vi "camera_number.vi"() -> ()   [LabVIEW 2022 SP3]
panel:
  in  "Refresh Button":bool
  in  "4 2":string
  in  "3 2":string caption="3"
  in  "2 2":string
  in  "1 2":string
  out "error out 8":errorcluster
  out "error out 7":errorcluster
  out "error out 6":errorcluster
  out "error out 5":errorcluster
  out "error out":errorcluster
  in  "OK Button 2":bool
  out "error out 2":errorcluster
  out "error out 3":errorcluster
  out "error out 4":errorcluster
  in  "4":string
  in  "3":string
  in  "2":string
  in  "1":string
  # "REFERENCE CHECK"
  # "CAM A"
  # "CAM B"
  # "CAM C"
  # "CAM D"
  # "Refresh"
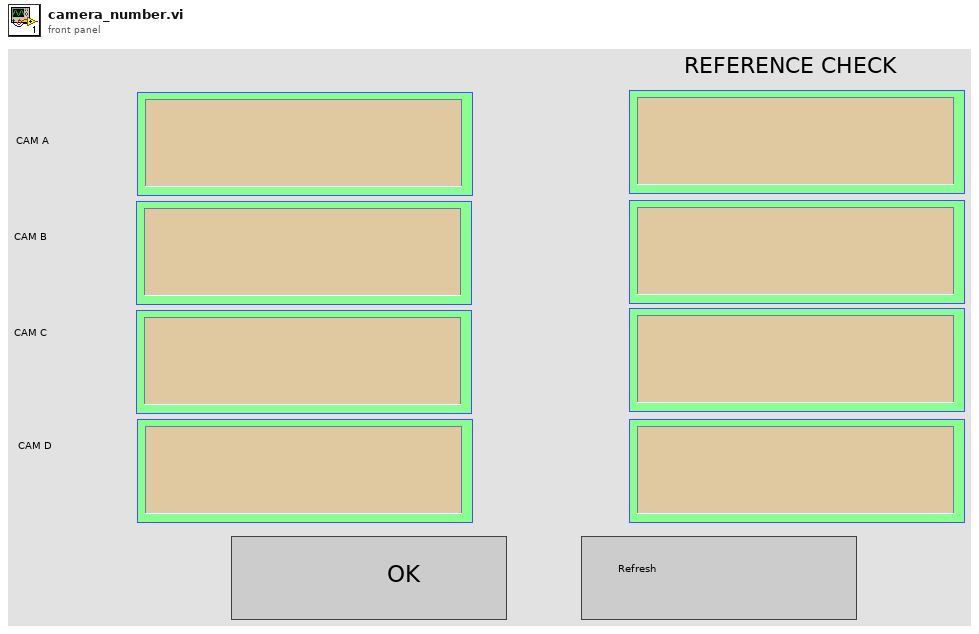
[diagram p1: front panel]
types:
  T1 = enum16{"open", "replace", "create", "open or create", "replace or create", "replace or create with confirmation"}
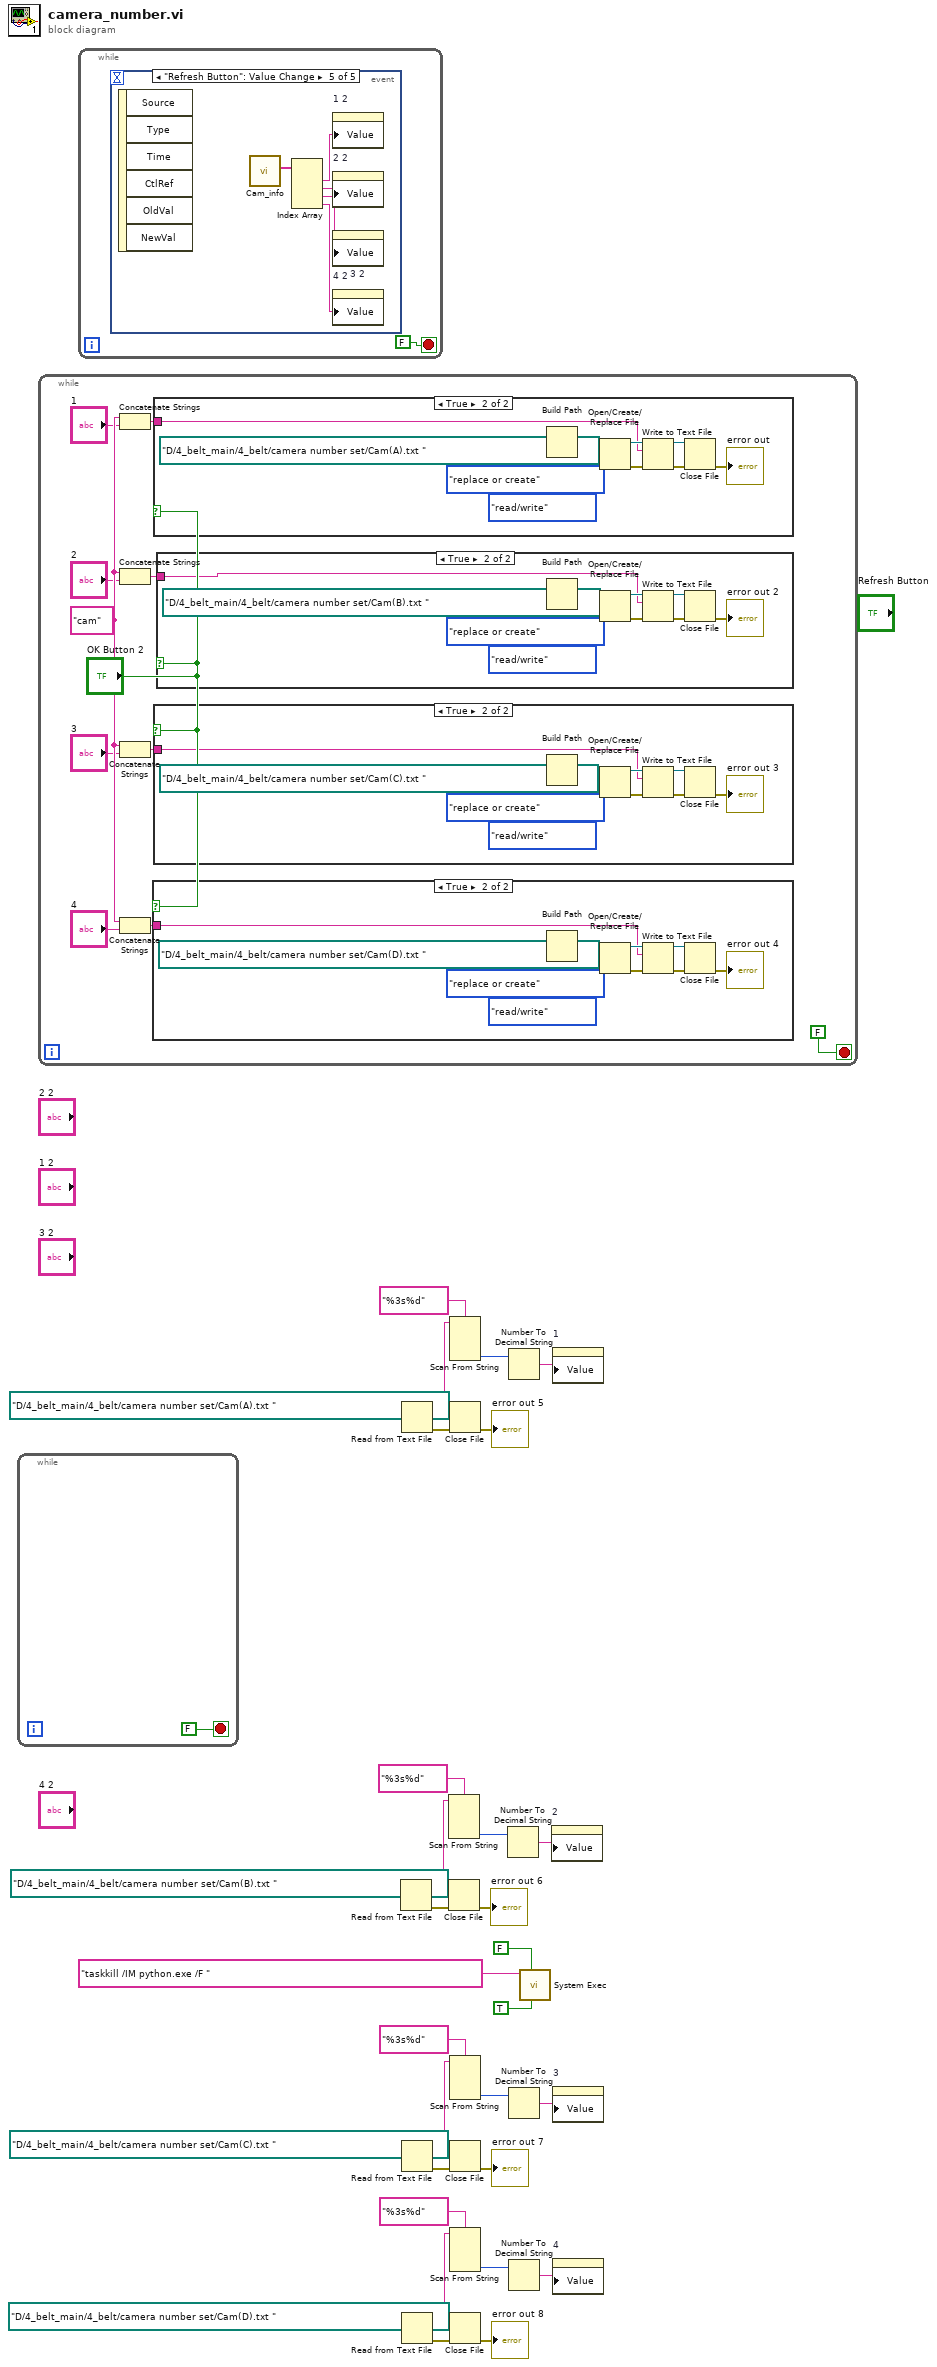
[diagram p0: block diagram]
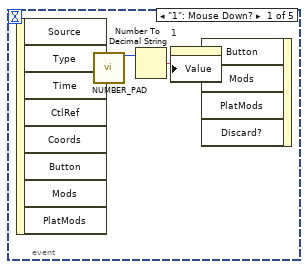
[diagram p2: hidden frame]
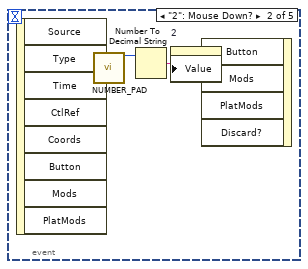
[diagram p3: hidden frame]
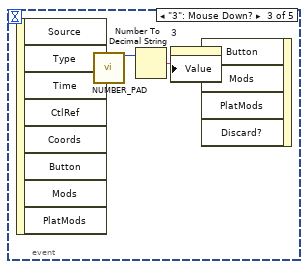
[diagram p4: hidden frame]
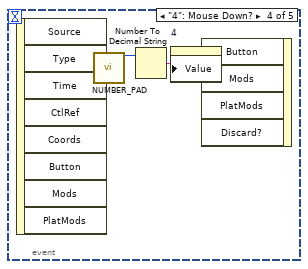
[diagram p5: hidden frame]
diagram:
  n1 = while {
    stop <- FALSE stop-if-true
  }
  n2 = while {
    stop <- FALSE stop-if-true
    w47 = "cam"
    n3 = Concatenate Strings(w47, "1") -> (w46:string)
    n4 = Concatenate Strings(w47, "2") -> (w45:string)
    n5 = Concatenate Strings(w47, "3") -> (w44:string)
    n6 = Concatenate Strings(w47, "4") -> (w43:string)
    n7 = case shown="True" "OK Button 2" {
      tunnel: w43 -> [_ w49]
      frame False {
      }
      frame True {
        n8 = Build Path(name or relative path=path "D:/4_belt_main/4_belt/camera number set/Cam(D).txt " ("base path")) -> (appended path=w57:path)  [unwired: 1 in]
        n9 = Open/Create/Replace File(file path (use dialog)=w57, operation (0:open)=T1."replace or create", access (0:read/write)=enum16{"read/write", "read-only", "write-only"}."read/write") -> (refnum out=w54:refnum<file>, error out=w53:errorcluster)  [unwired: 3 in, 1 out]
        n10 = Write to Text File(file (use dialog)=w54, text=w49, error in=w53) -> (refnum out=w51:refnum<file>, error out=w52:errorcluster)  [unwired: 1 in, 1 out]
        n11 = Close File(refnum=w51, error in=w52) -> (error out=→"error out 4":errorcluster)  [unwired: 1 out]
      }
    }
    n12 = case shown="True" "OK Button 2" {
      tunnel: w46 -> [_ w79]
      frame False {
      }
      frame True {
        n13 = Build Path(name or relative path=path "D:/4_belt_main/4_belt/camera number set/Cam(A).txt " ("base path")) -> (appended path=w87:path)  [unwired: 1 in]
        n14 = Open/Create/Replace File(file path (use dialog)=w87, operation (0:open)=T1."replace or create", access (0:read/write)=enum16{"read/write", "read-only", "write-only"}."read/write") -> (refnum out=w84:refnum<file>, error out=w83:errorcluster)  [unwired: 3 in, 1 out]
        n15 = Write to Text File(file (use dialog)=w84, text=w79, error in=w83) -> (refnum out=w81:refnum<file>, error out=w82:errorcluster)  [unwired: 1 in, 1 out]
        n16 = Close File(refnum=w81, error in=w82) -> (error out=→"error out":errorcluster)  [unwired: 1 out]
      }
    }
    n17 = case shown="True" "OK Button 2" {
      tunnel: w44 -> [_ w59]
      frame False {
      }
      frame True {
        n18 = Build Path(name or relative path=path "D:/4_belt_main/4_belt/camera number set/Cam(C).txt " ("base path")) -> (appended path=w67:path)  [unwired: 1 in]
        n19 = Open/Create/Replace File(file path (use dialog)=w67, operation (0:open)=T1."replace or create", access (0:read/write)=enum16{"read/write", "read-only", "write-only"}."read/write") -> (refnum out=w64:refnum<file>, error out=w63:errorcluster)  [unwired: 3 in, 1 out]
        n20 = Write to Text File(file (use dialog)=w64, text=w59, error in=w63) -> (refnum out=w61:refnum<file>, error out=w62:errorcluster)  [unwired: 1 in, 1 out]
        n21 = Close File(refnum=w61, error in=w62) -> (error out=→"error out 3":errorcluster)  [unwired: 1 out]
      }
    }
    n22 = case shown="True" "OK Button 2" {
      tunnel: w45 -> [_ w69]
      frame False {
      }
      frame True {
        n23 = Build Path(name or relative path=path "D:/4_belt_main/4_belt/camera number set/Cam(B).txt " ("base path")) -> (appended path=w77:path)  [unwired: 1 in]
        n24 = Open/Create/Replace File(file path (use dialog)=w77, operation (0:open)=T1."replace or create", access (0:read/write)=enum16{"read/write", "read-only", "write-only"}."read/write") -> (refnum out=w74:refnum<file>, error out=w73:errorcluster)  [unwired: 3 in, 1 out]
        n25 = Write to Text File(file (use dialog)=w74, text=w69, error in=w73) -> (refnum out=w71:refnum<file>, error out=w72:errorcluster)  [unwired: 1 in, 1 out]
        n26 = Close File(refnum=w71, error in=w72) -> (error out=→"error out 2":errorcluster)  [unwired: 1 out]
      }
    }
  }
  n27 = while {
    stop <- FALSE stop-if-true
    n28 = event shown="[4] \"Refresh Button\": Value Change" {
      selector: _ -> [_ _ _ _ _]
      dyn-events: _ -> [_ _ _ _ _]
      timeout: _ -> [_ _ _ _ _]
      event "1": Mouse Down? {
        n29 = event-data() -> ()  [unwired: 1 in, 8 out]
        n30 = call "NUMBER_PAD.vi"() -> ("number (out)"=w90:i32)  [unwired: 15 in]
        n31 = Number To Decimal String(number=w90) -> (decimal integer string=w89:string)  [unwired: 1 in]
        n32 = property on="1" class="Str"("Value"=w89) -> ()  [unwired: 2 in, 2 out]
        n33 = event-data() -> ()  [unwired: 5 in, 1 out]
      }
      event "2": Mouse Down? {
        n34 = event-data() -> ()  [unwired: 1 in, 8 out]
        n35 = call "NUMBER_PAD.vi"() -> ("number (out)"=w92:i32)  [unwired: 15 in]
        n36 = Number To Decimal String(number=w92) -> (decimal integer string=w91:string)  [unwired: 1 in]
        n37 = property on="2" class="Str"("Value"=w91) -> ()  [unwired: 2 in, 2 out]
        n38 = event-data() -> ()  [unwired: 5 in, 1 out]
      }
      event "3": Mouse Down? {
        n39 = event-data() -> ()  [unwired: 1 in, 8 out]
        n40 = call "NUMBER_PAD.vi"() -> ("number (out)"=w94:i32)  [unwired: 15 in]
        n41 = Number To Decimal String(number=w94) -> (decimal integer string=w93:string)  [unwired: 1 in]
        n42 = property on="3" class="Str"("Value"=w93) -> ()  [unwired: 2 in, 2 out]
        n43 = event-data() -> ()  [unwired: 5 in, 1 out]
      }
      event "4": Mouse Down? {
        n44 = event-data() -> ()  [unwired: 1 in, 8 out]
        n45 = call "NUMBER_PAD.vi"() -> ("number (out)"=w96:i32)  [unwired: 15 in]
        n46 = Number To Decimal String(number=w96) -> (decimal integer string=w95:string)  [unwired: 1 in]
        n47 = property on="4" class="Str"("Value"=w95) -> ()  [unwired: 2 in, 2 out]
        n48 = event-data() -> ()  [unwired: 5 in, 1 out]
      }
      event "Refresh Button": Value Change {
        n49 = event-data() -> ()  [unwired: 1 in, 6 out]
        n50 = call "Cam_info.vi"() -> ("All Cameras"=w101:string[])  [unwired: 10 in, 1 out]
        n51 = Index Array(array=w101) -> (element #1=w100:string, element #2=w99:string, element #3=w98:string, element #4=w97:string)  [unwired: 4 in]
        n52 = property on="1 2" class="Str"("Value"=w100) -> ()  [unwired: 2 in, 2 out]
        n53 = property on="2 2" class="Str"("Value"=w99) -> ()  [unwired: 2 in, 2 out]
        n54 = property on="3 2" class="Str"("Value"=w98) -> ()  [unwired: 2 in, 2 out]
        n55 = property on="4 2" class="Str"("Value"=w97) -> ()  [unwired: 2 in, 2 out]
      }
    }
  }
  n56 = Read from Text File(file (use dialog)=path "D:/4_belt_main/4_belt/camera number set/Cam(B).txt " ("base path")) -> (refnum out=w22:refnum<file>, text=w26:string, error out=w23:errorcluster)  [unwired: 3 in, 1 out]
  n57 = Read from Text File(file (use dialog)=path "D:/4_belt_main/4_belt/camera number set/Cam(A).txt " ("base path")) -> (refnum out=w35:refnum<file>, text=w31:string, error out=w34:errorcluster)  [unwired: 3 in, 1 out]
  n58 = Read from Text File(file (use dialog)=path "D:/4_belt_main/4_belt/camera number set/Cam(C).txt " ("base path")) -> (refnum out=w21:refnum<file>, text=w17:string, error out=w20:errorcluster)  [unwired: 3 in, 1 out]
  n59 = Read from Text File(file (use dialog)=path "D:/4_belt_main/4_belt/camera number set/Cam(D).txt " ("base path")) -> (refnum out=w8:refnum<file>, text=w12:string, error out=w9:errorcluster)  [unwired: 3 in, 1 out]
  n60 = Scan From String(format string="%3s%d", input string=w26) -> (output 2=w28:i32)  [unwired: 5 in, 3 out]
  n61 = Close File(refnum=w22, error in=w23) -> (error out=→"error out 6":errorcluster)  [unwired: 1 out]
  n62 = Scan From String(format string="%3s%d", input string=w31) -> (output 2=w29:i32)  [unwired: 5 in, 3 out]
  n63 = Close File(refnum=w35, error in=w34) -> (error out=→"error out 5":errorcluster)  [unwired: 1 out]
  n64 = Scan From String(format string="%3s%d", input string=w17) -> (output 2=w15:i32)  [unwired: 5 in, 3 out]
  n65 = Close File(refnum=w21, error in=w20) -> (error out=→"error out 7":errorcluster)  [unwired: 1 out]
  n66 = Scan From String(format string="%3s%d", input string=w12) -> (output 2=w14:i32)  [unwired: 5 in, 3 out]
  n67 = Close File(refnum=w8, error in=w9) -> (error out=→"error out 8":errorcluster)  [unwired: 1 out]
  n68 = Number To Decimal String(number=w28) -> (decimal integer string=w2:string)  [unwired: 1 in]
  n69 = Number To Decimal String(number=w29) -> (decimal integer string=w1:string)  [unwired: 1 in]
  n70 = Number To Decimal String(number=w15) -> (decimal integer string=w3:string)  [unwired: 1 in]
  n71 = Number To Decimal String(number=w14) -> (decimal integer string=w4:string)  [unwired: 1 in]
  n72 = call <vilib>:"System Exec.vi"("run minimized? (F)"=TRUE, "wait until completion? (T)"=FALSE, "command line"="taskkill /IM python.exe /F ") -> ()  [unwired: 5 in, 4 out]
  n73 = property on="2" class="Str"("Value"=w2) -> ()  [unwired: 2 in, 2 out]
  n74 = property on="1" class="Str"("Value"=w1) -> ()  [unwired: 2 in, 2 out]
  n75 = property on="3" class="Str"("Value"=w3) -> ()  [unwired: 2 in, 2 out]
  n76 = property on="4" class="Str"("Value"=w4) -> ()  [unwired: 2 in, 2 out]
